vi "Configure Heater Outputs.vi"(0 "VISA resource name":refnum<visa-resource-name>, 1 "Heater Output (1:1)":u16(ring)=1 items=["1"=1, "2"=2], 2 "Mode (0:Off)":u16(ring) items=["Off", "Closed Loop PID", "Zone", "Open Loop", "Monitor Out", "Warmup Supply"], 3 "Max Current (0:User Specified)":u16(ring) items=["User Specified", "0.707 A", "1.0 A", "1.141 A", "1.732 A"], 4 "Max User Current (1.732)":dbl=1.732 format="%.3f", 5 "error in (no error)":errorcluster, 6 "Input (0:None)":u16(ring) items=["None", "A", "B"], 7 "Heater Out Display (1:Current)":u16(ring)=1 items=["Current"=1, "Power"=2], 8 "Heater Resistance (1:25 Ohm)":u16(ring)=1 items=["25 Ohm"=1, "50 Ohm"=2], 9 "Polarity (0:Unipolar)":u16(ring) items=["Unipolar", "Bipolar"], 10 "Power Up Enable (F: Off)":bool, 11 "Output Type (0:Current)":u16(ring) items=["Current", "Voltage"]) -> (14 "VISA resource name out":refnum<visa-resource-name>, 19 "error out":errorcluster)   [LabVIEW 2015, in "Lake Shore 335.lvlib"]
doc: "Configures the heater outputs. Heater Outputs 1 and 2 are traditional control loop heater outputs for a cryogenic temperature controller. The two outputs are identical except in the amount of power available. Output 1 can provide up to 75 W when Output 2 is configured as a voltage output, or 50 W when Output 2 is configured as a current output. Output 2 can provide up to 25 W when configured as a current output, and 1 W when it is configured as a voltage output."
uses:
  <instrlib>/Lake Shore 335/Lake Shore 335.lvlib
  <instrlib>/Lake Shore 335/Private/Extended User Data.ctl
panel:
  # "Settings for Either Heater Output"
  # "Settings for Heater Output 2 Only"
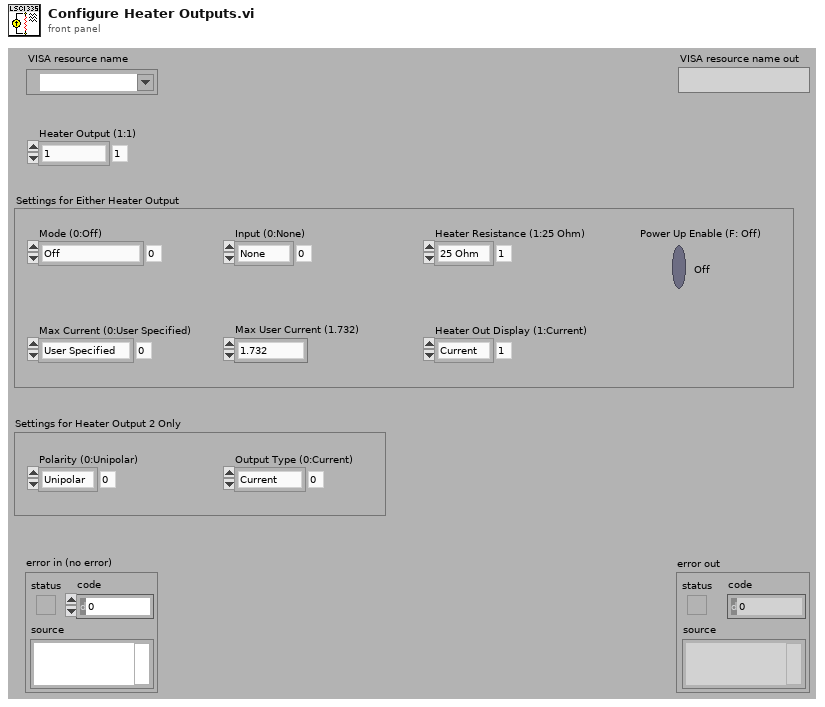
[diagram p1: front panel]
types:
  T1 = typedef "Lake Shore 335.lvlib/Extended User Data.ctl" = cluster{"Mode (0:Off)":u16, "Polarity (0:Unipolar)":u16, "Output Type (0:Current)":u16, "Input (0:None)":u16}
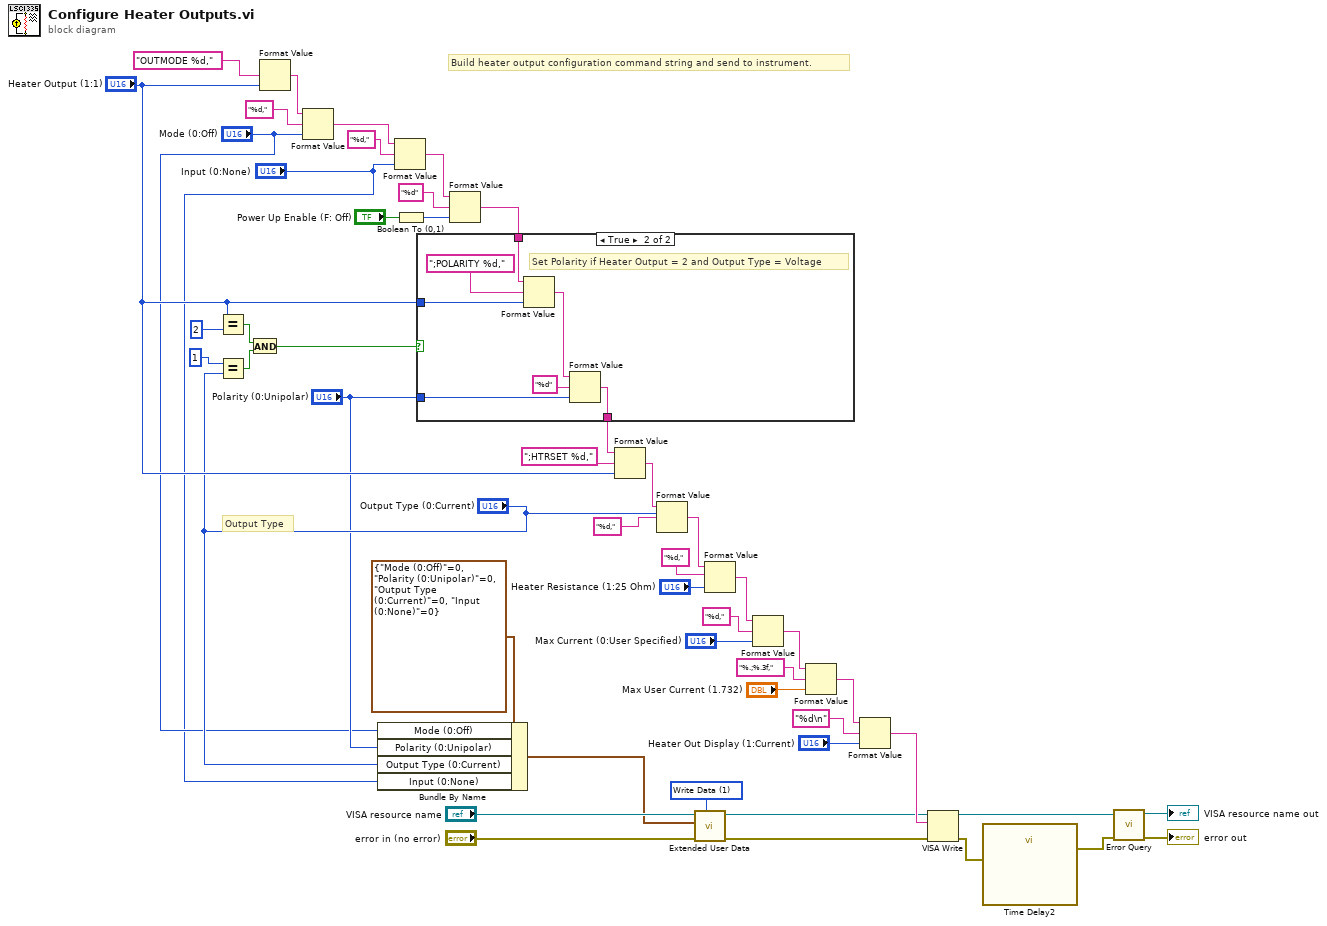
[diagram p0: block diagram]
diagram:
  w8 = u16 1 items=["Read Data", "Write Data", "Clear Data", "Clear ALL Data"] ("Action")
  # "Output Type"
  # "Build heater output configuration command string and send to instrument."
  n1 = Equal?(x="Heater Output (1:1)", y=u16 2) -> (x = y?=w17:bool)
  n2 = Equal?(x=u16 1, y="Output Type (0:Current)") -> (x = y?=w16:bool)
  n3 = And(x=w17, y=w16) -> (x .and. y?=w15:bool)
  n4 = Format Value(format string="OUTMODE %d,", value (0)="Heater Output (1:1)") -> (output string=w25:string)  [unwired: 1 in]
  n5 = Format Value(string ("")=w25, format string="%d,", value (0)="Mode (0:Off)") -> (output string=w33:string)
  n6 = Bundle By Name(cluster=T1 {"Mode (0:Off)"=0, "Polarity (0:Unipolar)"=0, "Output Type (0:Current)"=0, "Input (0:None)"=0} ("User Data Definition"), "Mode (0:Off)"="Mode (0:Off)", "Polarity (0:Unipolar)"="Polarity (0:Unipolar)", "Output Type (0:Current)"="Output Type (0:Current)", "Input (0:None)"="Input (0:None)") -> (w3:T1)
  n7 = Format Value(string ("")=w33, format string="%d,", value (0)="Input (0:None)") -> (output string=w32:string)
  n8 = Boolean To (0,1)(Boolean="Power Up Enable (F: Off)") -> (0, 1=w45:i16)
  n9 = Format Value(string ("")=w32, format string="%d", value (0)=w45) -> (output string=w14:string)
  n10 = case shown="True" w15 {
    tunnel: w14 -> [w50 w56]
    tunnel: "Heater Output (1:1)" -> [_ w55]
    tunnel: [w50 w52] -> w13
    tunnel: "Polarity (0:Unipolar)" -> [_ w51]
    frame False {
      # "Do not set Polarity"
    }
    frame True {
      # "Set Polarity if Heater Output = 2 and Output Type = Voltage"
      n11 = Format Value(string ("")=w56, format string=";POLARITY %d,", value (0)=w55) -> (output string=w53:string)
      n12 = Format Value(string ("")=w53, format string="%d", value (0)=w51) -> (output string=w52:string)
    }
  }
  n13 = Format Value(string ("")=w13, format string=";HTRSET %d,", value (0)="Heater Output (1:1)") -> (output string=w20:string)
  n14 = Format Value(string ("")=w20, format string="%d,", value (0)="Output Type (0:Current)") -> (output string=w21:string)
  n15 = call <instrlib>:"Extended User Data.vi"("Action"=w8, "Error In (no error)"="error in (no error)", "User Data In"=w3, "VISA resource name in"="VISA resource name") -> ("Error Out"=w9:errorcluster, "VISA resource name out"=w10:refnum<visa-resource-name>)  [unwired: 5 in, 1 out]
  n16 = Format Value(string ("")=w21, format string="%d,", value (0)="Heater Resistance (1:25 Ohm)") -> (output string=w31:string)
  n17 = Format Value(string ("")=w31, format string="%d,", value (0)="Max Current (0:User Specified)") -> (output string=w38:string)
  n18 = Format Value(string ("")=w38, format string="%.;%.3f,", value (0)="Max User Current (1.732)") -> (output string=w30:string)
  n19 = Format Value(string ("")=w30, format string="%d\n", value (0)="Heater Out Display (1:Current)") -> (output string=w26:string)
  n20 = VISA Write(VISA resource name=w10, write buffer=w26, error in (no error)=w9) -> (VISA resource name out=w27:refnum<visa-resource-name>, error out=w29:errorcluster)  [unwired: 1 out]
  n21 = call "Time Delay2"("error in (no error)"=w29) -> ("error out"=w28:errorcluster)  [unwired: 10 in]
  n22 = call <instrlib>:"Error Query.vi"("error in (no error)"=w28, "VISA resource name"=w27) -> ("error out"=→"error out":errorcluster, "VISA resource name out"=→"VISA resource name out":refnum<visa-resource-name>)  [unwired: 7 in, 1 out]
